vi "Menu.Sequence.Load.vi"(8 "error in (no error)":errorcluster, 9 "Coords":T1, 10 "MenuRef":refnum<k9>, 11 "State Variables":T2={"Aliases.All"=[], "Aliases.Outputs"=[], "UI.Sequence#ofColumns"=0, "SysDef.Path"=path "", "UI.SequenceRef"=refnum, "UI.StepInformationRef"=refnum, "UI.AbortRef"=refnum, "UI.GraphRef"=refnum, "UI.ViewRef"=refnum, "UI.IterationsRef"=refnum, "UI.IterationInformationRef"=refnum, "INI.Settings"={"Build Location"=path "C:/Simple Sequence Editor/SequenceRepo", "LoggingLocation"=path ""}}) -> (0 "error out":errorcluster, 3 "State Variables out":T2={"Aliases.All"=[], "Aliases.Outputs"=[], "UI.Sequence#ofColumns"=0, "SysDef.Path"=path "", "UI.SequenceRef"=refnum, "UI.StepInformationRef"=refnum, "UI.AbortRef"=refnum, "UI.GraphRef"=refnum, "UI.ViewRef"=refnum, "UI.IterationsRef"=refnum, "UI.IterationInformationRef"=refnum, "INI.Settings"={"Build Location"=path "C:/Simple Sequence Editor/SequenceRepo", "LoggingLocation"=path ""}})   [LabVIEW 2013, in "Simple Sequence Tools - Editor.lvlib"]
uses:
  Simple Sequence Tools - Editor.lvlib
  Types/StateVariables.ctl
  Shared/Types/ChannelProperties.ctl
  Shared/Types/INI.Settings
  <vilib>/Utility/miscctls.llb/LVPoint32TypeDef.ctl
  Shared/SubVIs/Constants.vi
  Shared/Simple Sequence Tools - Shared.lvlib
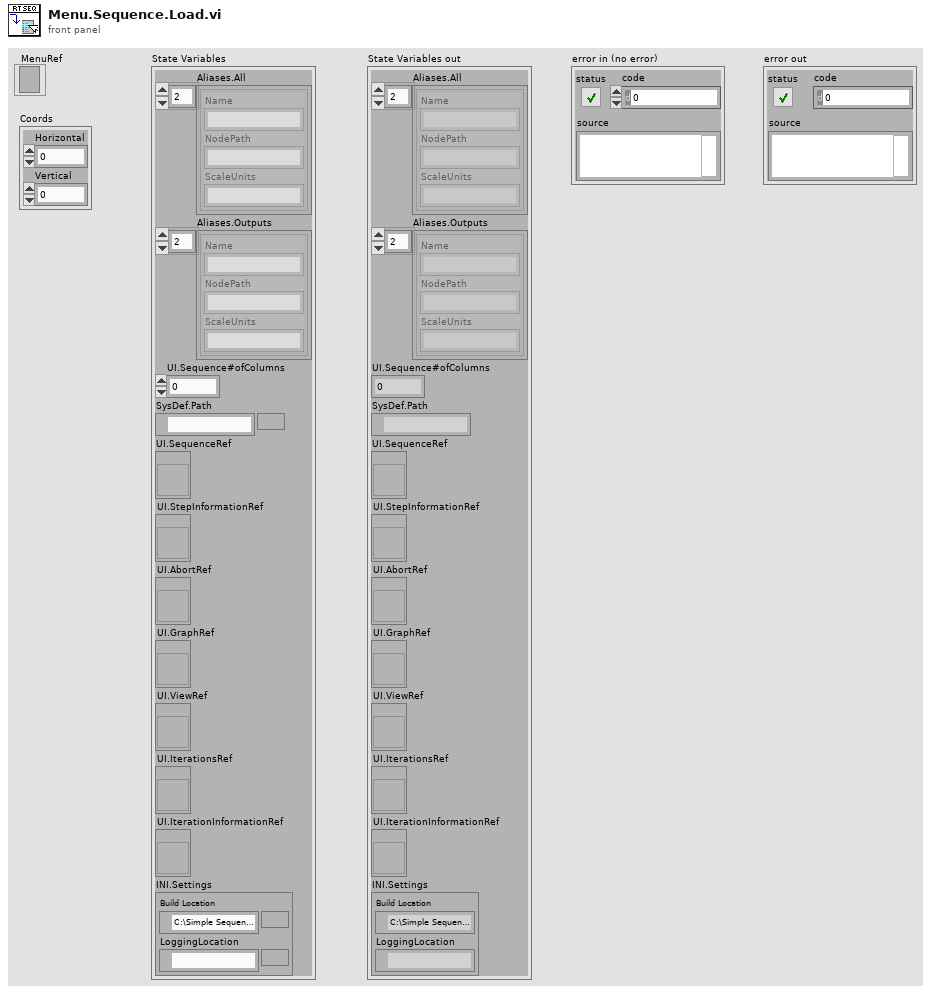
[diagram p1: front panel]
types:
  T1 = typedef "LVPoint32TypeDef.ctl" = cluster{"Horizontal":i32, "Vertical":i32}
  T2 = typedef "Simple Sequence Tools - Editor.lvlib/StateVariables.ctl" = cluster{"Aliases.All":T3[], "Aliases.Outputs":T3[], "UI.Sequence#ofColumns":i32, "SysDef.Path":path, "UI.SequenceRef":refnum<vi>, "UI.StepInformationRef":refnum<vi>, "UI.AbortRef":refnum<vi>, "UI.GraphRef":refnum<vi>, "UI.ViewRef":refnum<vi>, "UI.IterationsRef":refnum<vi>, "UI.IterationInformationRef":refnum<vi>, "INI.Settings":T4}
  T3 = typedef "Simple Sequence Tools - Shared.lvlib/ChannelProperties.ctl" = cluster{"Name":string, "NodePath":string, "ScaleUnits":string}
  T4 = typedef "Simple Sequence Tools - Shared.lvlib/INI.Settings" = cluster{"Build Location":path, "LoggingLocation":path}
  T5 = typedef "LVRowAndColumnTypeDef.ctl" = cluster{"Row":i32, "Column":i32}
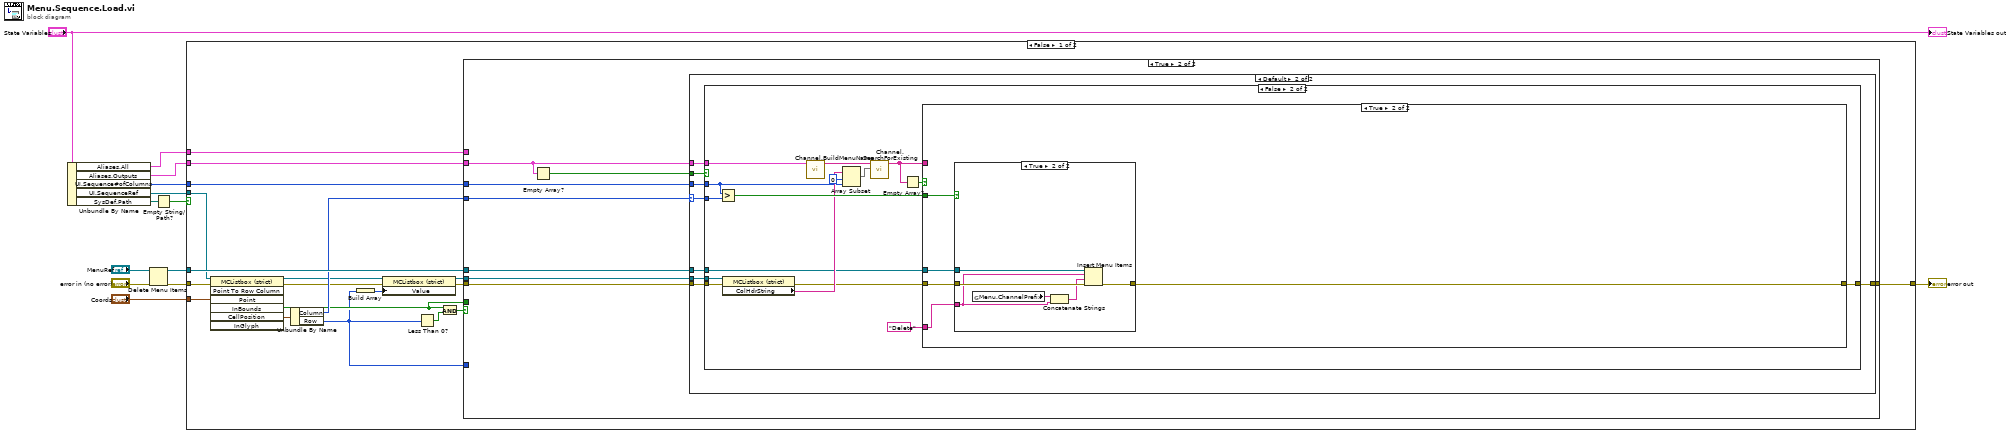
[diagram p0: block diagram]
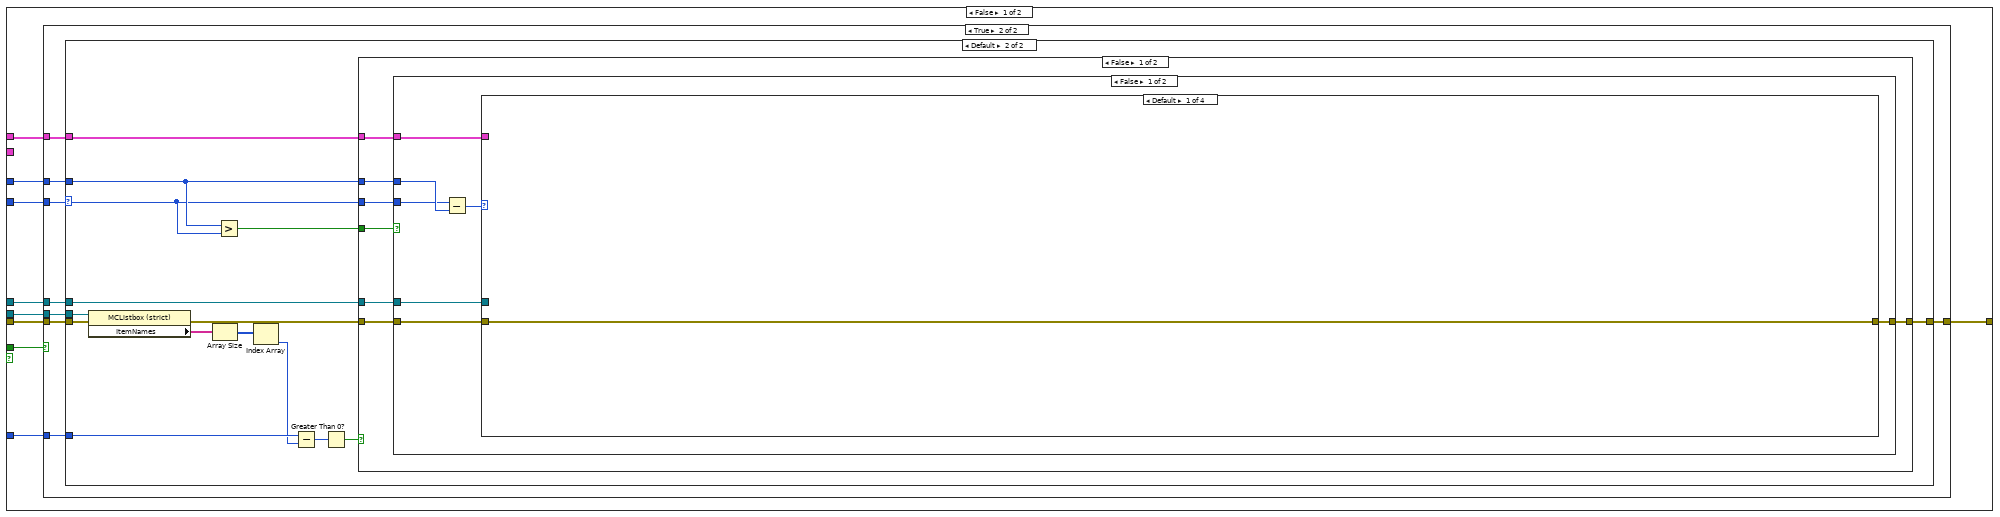
[diagram p2: hidden frame]
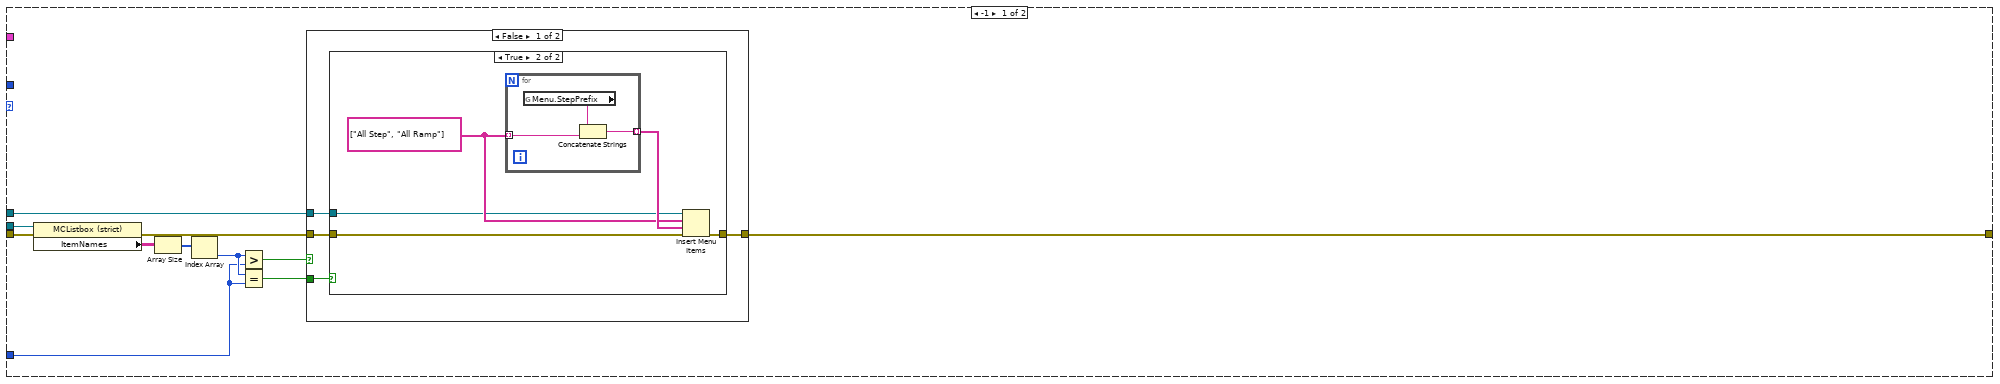
[diagram p4: hidden frame]
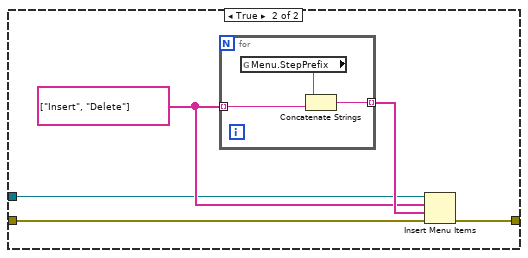
[diagram p6: hidden frame]
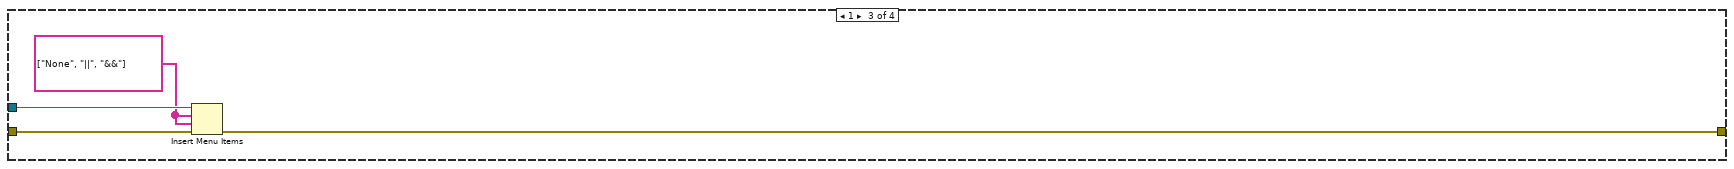
[diagram p8: hidden frame]
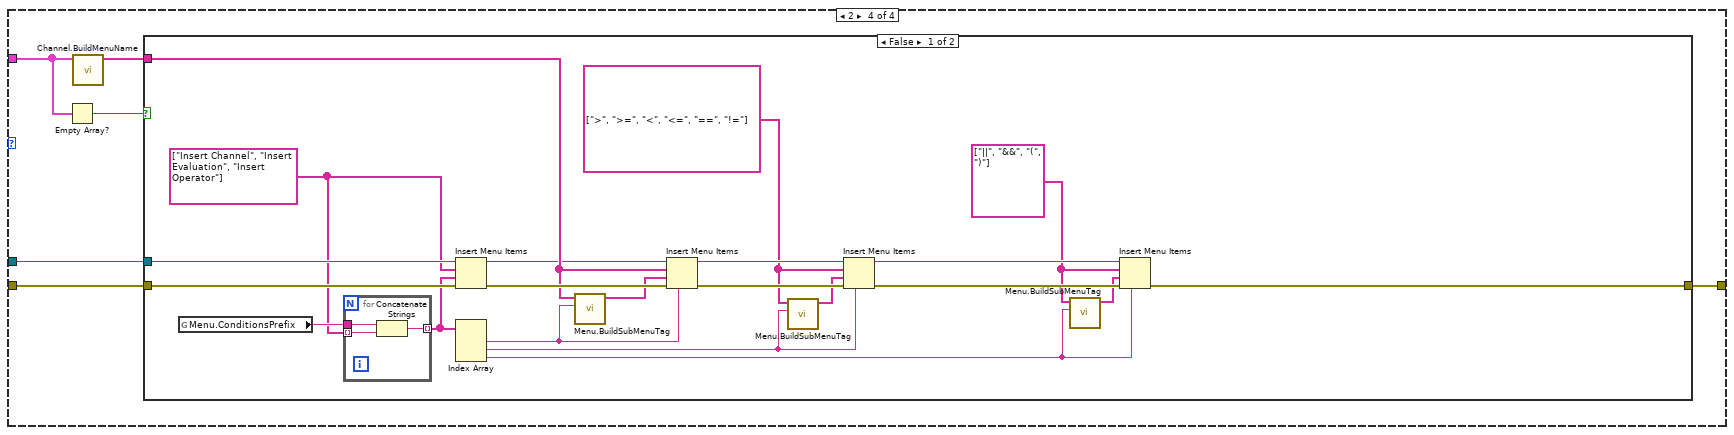
[diagram p9: hidden frame]
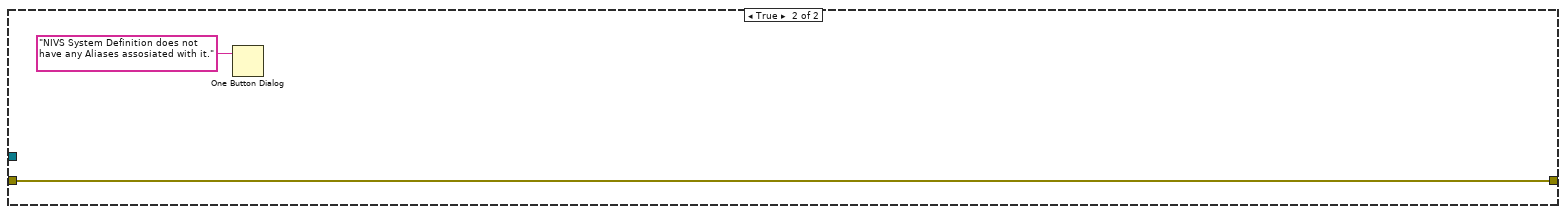
[diagram p10: hidden frame]
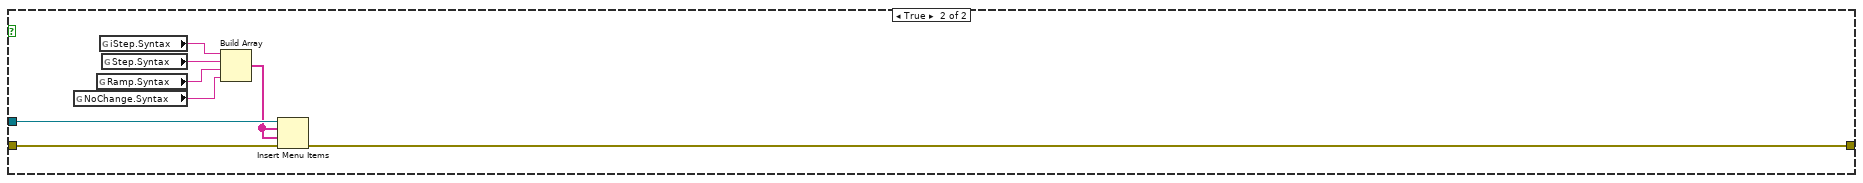
[diagram p11: hidden frame]
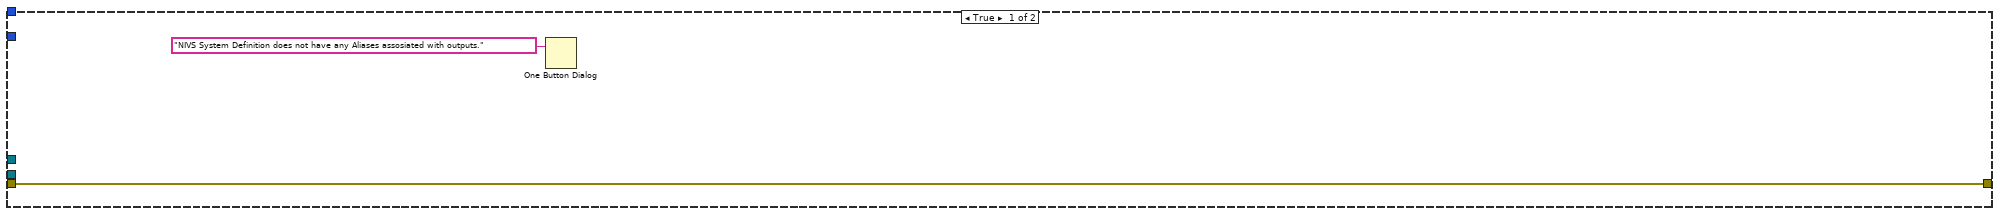
[diagram p14: hidden frame]
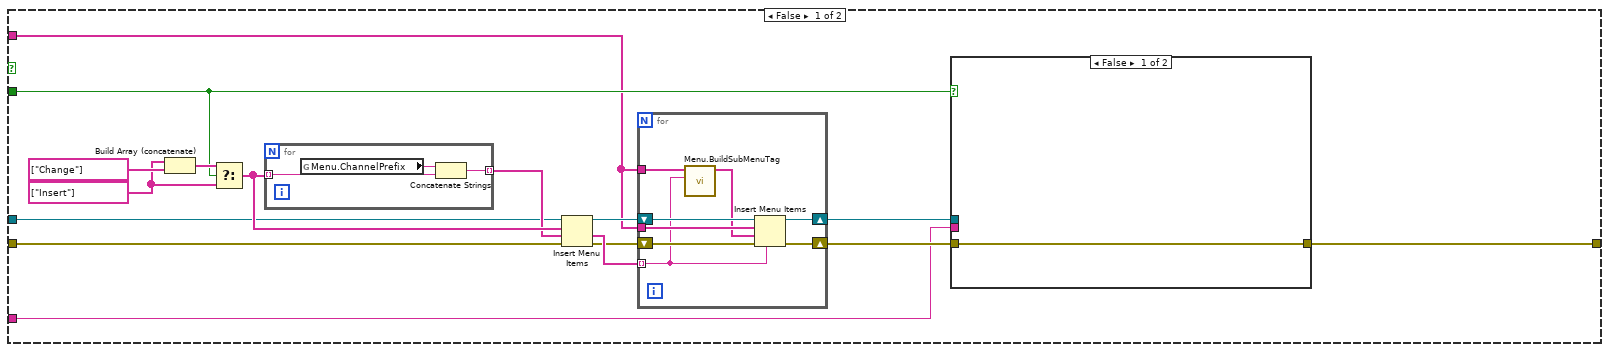
[diagram p15: hidden frame]
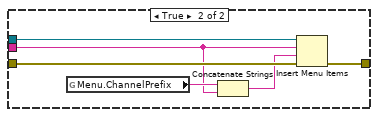
[diagram p16: hidden frame]
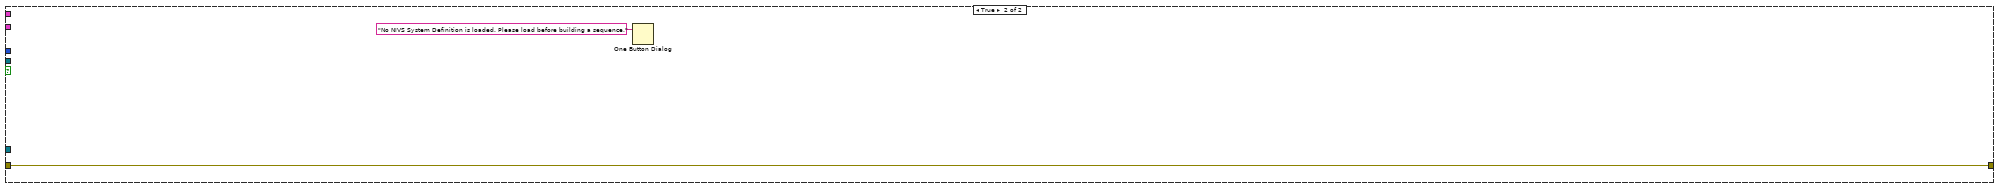
[diagram p18: hidden frame]
diagram:
  n1 = Unbundle By Name("State Variables") -> ("Aliases.All"=w1:T3[], "Aliases.Outputs"=w9:T3[], "UI.Sequence#ofColumns"=w12:i32, "UI.SequenceRef"=w10:refnum<vi>, "SysDef.Path"=w7:path)
  n2 = Delete Menu Items(6:"error in (no error)", 9:"MenuRef") -> (0:w4:errorcluster, 3:w2:refnum<k9>)  [unwired: 2 in]
  n3 = Empty String/Path?(string/path=w7) -> (empty?=w6:bool)
  n4 = case shown="False" w6 {
    tunnel: [w32 w240] -> w13
    tunnel: w2 -> [w31 _]
    tunnel: w12 -> [w30 _]
    tunnel: "Coords" -> [w25 _]
    tunnel: w10 -> [w24 _]
    tunnel: w4 -> [w23 w240]
    tunnel: w9 -> [w22 _]
    tunnel: w1 -> [w20 _]
    frame False {
      n5 = invoke class="MCListbox (strict)" method="Point To Row Column"(reference=w24, error in=w23, "Point"=w25) -> (reference out=w18:refnum<vi>, error out=w19:errorcluster, "InBounds"=w21:bool, "CellPosition"=w26:T5)  [unwired: 4 in, 3 out]
      n6 = Unbundle By Name(w26) -> ("Column"=w29:i32, "Row"=w15:i32)
      n7 = Build Array(w15) -> (w14:i32[])
      n8 = property class="MCListbox (strict)"(reference=w18, error in=w19, "Value"=w14) -> (reference out=w16:refnum<vi>, error out=w17:errorcluster)
      n9 = Less Than 0?(x=w15) -> (x < 0?=w27:bool)
      n10 = And(x=w21, y=w27) -> (x .and. y?=w28:bool)
      n11 = case shown="True" w28 {
        tunnel: w29 -> [w36 w159]
        tunnel: w30 -> [w37 w160]
        tunnel: w31 -> [w35 w163]
        tunnel: w17 -> [w40 w164]
        tunnel: [w34 w165] -> w32
        tunnel: w16 -> [w39 w166]
        tunnel: w22 -> [_ w162]
        tunnel: w21 -> [w41 _]
        tunnel: w15 -> [w38 _]
        tunnel: w20 -> [w33 _]
        frame False {
          n12 = case shown="True" w41 {
            tunnel: w40 -> [w42 w49]
            tunnel: w39 -> [_ w50]
            tunnel: w38 -> [_ w48]
            tunnel: w37 -> [_ w47]
            tunnel: w36 -> [_ w46]
            tunnel: w35 -> [_ w45]
            tunnel: [w42 w44] -> w34
            tunnel: w33 -> [_ w43]
            frame False {
            }
            frame True {
              n13 = case shown="Default" w46 {
                selector: w46 -> [_ w87]
                tunnel: w50 -> [w57 w97]
                tunnel: w49 -> [w59 w96]
                tunnel: w48 -> [w52 w93]
                tunnel: w47 -> [_ w88]
                tunnel: w45 -> [w60 w89]
                tunnel: [w61 w85] -> w44
                tunnel: w43 -> [_ w83]
                frame -1 {
                  n14 = property class="MCListbox (strict)"(reference=w57, error in=w59) -> (error out=w58:errorcluster, "ItemNames"=w55:string[][])  [unwired: 1 out]
                  n15 = Array Size(array=w55) -> (size(s)=w56:i32[])
                  n16 = Index Array(array=w56) -> (element=w53:i32)  [unwired: 1 in]
                  n17 = Greater?(x=w53, y=w52) -> (0:w54:bool)
                  n18 = Equal?(x=w53, y=w52) -> (x = y?=w51:bool)
                  n19 = case shown="False" w54 {
                    tunnel: [w64 w79] -> w61
                    tunnel: w60 -> [w63 w76]
                    tunnel: w58 -> [w65 w75]
                    tunnel: w51 -> [w62 _]
                    frame False {
                      n20 = case shown="True" w62 {
                        tunnel: w65 -> [w66 w69]
                        tunnel: [w66 w68] -> w64
                        tunnel: w63 -> [_ w67]
                        frame False {
                        }
                        frame True {
                          w70 = string[] ["All Step", "All Ramp"] ("item names")
                          n21 = for {
                            tunnel: [w73] -> w71 mode=indexing
                            tunnel: w70 -> [w74] mode=indexing
                            n22 = global read "Constants.vi" "Menu.StepPrefix"() -> (w72:string)
                            n23 = Concatenate Strings(w72, w74) -> (w73:string)
                          }
                          n24 = Insert Menu Items(6:w69, 7:w71, 8:w70, 9:w67) -> (0:w68:errorcluster)  [unwired: 2 in, 2 out]
                        }
                      }
                    }
                    frame True {
                      w77 = string[] ["Insert", "Delete"] ("item names")
                      n25 = for {
                        tunnel: [w81] -> w78 mode=indexing
                        tunnel: w77 -> [w82] mode=indexing
                        n26 = global read "Constants.vi" "Menu.StepPrefix"() -> (w80:string)
                        n27 = Concatenate Strings(w80, w82) -> (w81:string)
                      }
                      n28 = Insert Menu Items(6:w75, 7:w78, 8:w77, 9:w76) -> (0:w79:errorcluster)  [unwired: 2 in, 2 out]
                    }
                  }
                }
                frame Default {
                  n29 = property class="MCListbox (strict)"(reference=w97, error in=w96) -> (error out=w91:errorcluster, "ItemNames"=w95:string[][])  [unwired: 1 out]
                  n30 = Array Size(array=w95) -> (size(s)=w94:i32[])
                  n31 = Greater?(x=w88, y=w87) -> (0:w86:bool)
                  n32 = Index Array(array=w94) -> (element=w92:i32)  [unwired: 1 in]
                  n33 = Subtract(x=w93, y=w92) -> (x-y=w84:i32)
                  n34 = Greater Than 0?(x=w84) -> (x > 0?=w90:bool)
                  n35 = case shown="False" w90 {
                    tunnel: w91 -> [w104 w158]
                    tunnel: w88 -> [w101 _]
                    tunnel: w87 -> [w100 _]
                    tunnel: w89 -> [w103 _]
                    tunnel: w86 -> [w102 _]
                    tunnel: [w99 w158] -> w85
                    tunnel: w83 -> [w98 _]
                    frame False {
                      n36 = case shown="False" w102 {
                        tunnel: w104 -> [w107 w157]
                        tunnel: w103 -> [w108 w155]
                        tunnel: w101 -> [w111 _]
                        tunnel: w100 -> [w110 _]
                        tunnel: [w106 w156] -> w99
                        tunnel: w98 -> [w105 _]
                        frame False {
                          n37 = Subtract(x=w110, y=w111) -> (x-y=w109:i32)
                          n38 = case shown="Default" w109 {
                            tunnel: w108 -> [_ _ w117 w123]
                            tunnel: w107 -> [w112 w113 w116 w122]
                            tunnel: [w112 w113 w114 w121] -> w106
                            tunnel: w105 -> [_ _ _ w120]
                            frame Default {
                            }
                            frame 0 {
                            }
                            frame 1 {
                              w115 = string[] ["None", "||", "&&"] ("item names")
                              n39 = Insert Menu Items(6:w116, 7:w115, 8:w115, 9:w117) -> (0:w114:errorcluster)  [unwired: 2 in, 2 out]
                            }
                            frame 2 {
                              n40 = Empty Array?(array=w120) -> (empty?=w119:bool)
                              n41 = call "Channel.BuildMenuName.vi"("Aliases"=w120) -> ("Aliases Array"=w118:string[])  [unwired: 10 in]
                              n42 = case shown="False" w119 {
                                tunnel: w123 -> [w144 _]
                                tunnel: w122 -> [w143 w148]
                                tunnel: [w132 w148] -> w121
                                tunnel: w118 -> [w138 _]
                                frame False {
                                w125 = string[] [">", ">=", "<", "<=", "==", "!="] ("item names")
                                w124 = string[] ["||", "&&", "(", ")"] ("item names")
                                w141 = string[] ["Insert Channel", "Insert Evaluation", "Insert Operator"] ("item names")
                                n43 = global read "Constants.vi" "Menu.ConditionsPrefix"() -> (w142:string)
                                n44 = for {
                                tunnel: w141 -> [w147] mode=indexing
                                tunnel: w142 -> [w146]
                                tunnel: [w145] -> w135 mode=indexing
                                n45 = Concatenate Strings(w146, w147) -> (w145:string)
                                }
                                n46 = Insert Menu Items(6:w143, 7:w135, 8:w141, 9:w144) -> (0:w140:errorcluster, 3:w137:refnum<k9>)  [unwired: 2 in, 1 out]
                                n47 = Index Array(array=w135) -> (element #1=w136:string, element #2=w129:string, element #3=w127:string)  [unwired: 3 in]
                                n48 = call "Menu.BuildSubMenuTag.vi"("Menu"=w136, "Aliases Array"=w138) -> ("Tag Array"=w139:string[])  [unwired: 9 in]
                                n49 = Insert Menu Items(5:w136, 6:w140, 7:w139, 8:w138, 9:w137) -> (0:w134:errorcluster, 3:w131:refnum<k9>)  [unwired: 1 in, 1 out]
                                n50 = call "Menu.BuildSubMenuTag.vi"("Menu"=w129, "Aliases Array"=w125) -> ("Tag Array"=w128:string[])  [unwired: 9 in]
                                n51 = Insert Menu Items(5:w129, 6:w134, 7:w128, 8:w125, 9:w131) -> (0:w133:errorcluster, 3:w130:refnum<k9>)  [unwired: 1 in, 1 out]
                                n52 = call "Menu.BuildSubMenuTag.vi"("Menu"=w127, "Aliases Array"=w124) -> ("Tag Array"=w126:string[])  [unwired: 9 in]
                                n53 = Insert Menu Items(5:w127, 6:w133, 7:w126, 8:w124, 9:w130) -> (0:w132:errorcluster)  [unwired: 1 in, 2 out]
                                }
                                frame True {
                                n54 = One Button Dialog(message="NIVS System Definition does not have any Aliases assosiated with it.") -> ()  [unwired: 1 in, 1 out]
                                }
                              }
                            }
                          }
                        }
                        frame True {
                          n55 = global read "Constants.vi" "NoChange.Syntax"() -> (w151:string)
                          n56 = global read "Constants.vi" "Ramp.Syntax"() -> (w153:string)
                          n57 = global read "Constants.vi" "iStep.Syntax"() -> (w150:string)
                          n58 = global read "Constants.vi" "Step.Syntax"() -> (w154:string)
                          n59 = Build Array(w150, w154, w153, w151) -> (w152:string[])
                          n60 = Insert Menu Items(6:w157, 7:w152, 8:w152, 9:w155) -> (0:w156:errorcluster)  [unwired: 2 in, 2 out]
                        }
                      }
                    }
                    frame True {
                    }
                  }
                }
              }
            }
          }
        }
        frame True {
          n61 = Empty Array?(array=w162) -> (empty?=w161:bool)
          n62 = case shown="Default" w159 {
            selector: w159 -> [_ w168]
            tunnel: w166 -> [_ w175]
            tunnel: [w167 w174] -> w165
            tunnel: w164 -> [w167 w173]
            tunnel: w163 -> [_ w172]
            tunnel: w162 -> [_ w171]
            tunnel: w161 -> [_ w170]
            tunnel: w160 -> [_ w169]
            frame -1 {
            }
            frame Default {
              n63 = case shown="False" w170 {
                tunnel: w168 -> [_ w193]
                tunnel: w175 -> [_ w191]
                tunnel: w169 -> [_ w189]
                tunnel: [w177 w187] -> w174
                tunnel: w171 -> [_ w186]
                tunnel: w173 -> [w177 w182]
                tunnel: w172 -> [_ w183]
                frame True {
                  n64 = One Button Dialog(message="NIVS System Definition does not have any Aliases assosiated with outputs.") -> ()  [unwired: 1 in, 1 out]
                }
                frame False {
                  n65 = Greater?(x=w189, y=w193) -> (0:w192:bool)
                  n66 = property class="MCListbox (strict)"(reference=w191, error in=w182) -> (error out=w181:errorcluster, "ColHdrString"=w190:string[])  [unwired: 1 out]
                  n67 = call "Channel.BuildMenuName.vi"("Aliases"=w186) -> ("Aliases Array"=w184:string[])  [unwired: 10 in]
                  n68 = Array Subset(array=w190, index=0, length=w189) -> (w185:string[])
                  n69 = call "Channel.SearchForExisting.vi"("Existing Channels"=w185, "All Channels"=w184) -> ("Array out"=w180:string[])  [unwired: 9 in]
                  n70 = Empty Array?(array=w180) -> (empty?=w179:bool)
                  n71 = case shown="True" w179 {
                    tunnel: w192 -> [w195 w228]
                    tunnel: [w198 w231] -> w187
                    tunnel: w183 -> [w202 w230]
                    tunnel: w180 -> [w194 _]
                    tunnel: w181 -> [w200 w232]
                    tunnel: "Delete" ("string") -> [w196 w229]
                    frame False {
                      w207 = string[] ["Insert"]
                      n72 = Build Array (concatenate)(w207, string[] ["Change"]) -> (w208:string[])
                      n73 = Select(t=w208, s=w195, f=w207) -> (s? t:f=w206:string[])
                      n74 = for {
                        tunnel: w206 -> [w227] mode=indexing
                        tunnel: [w226] -> w205 mode=indexing
                        n75 = global read "Constants.vi" "Menu.ChannelPrefix"() -> (w225:string)
                        n76 = Concatenate Strings(w225, w227) -> (w226:string)
                      }
                      n77 = Insert Menu Items(6:w200, 7:w205, 8:w206, 9:w202) -> (0:w201:errorcluster, 1:w203:string[], 3:w204:refnum<k9>)  [unwired: 2 in]
                      n78 = for {
                        tunnel: w203 -> [w219] mode=indexing
                        shift-right: [w223] -> w199
                        shift-left: w201 -> [w224]
                        tunnel: w194 -> [w221]
                        shift-right: [w220] -> w197
                        shift-left: w204 -> [w222]
                        tunnel: w194 -> [w218]
                        n79 = call "Menu.BuildSubMenuTag.vi"("Menu"=w219, "Aliases Array"=w218) -> ("Tag Array"=w217:string[])  [unwired: 9 in]
                        n80 = Insert Menu Items(5:w219, 6:w224, 7:w217, 8:w221, 9:w222) -> (0:w223:errorcluster, 3:w220:refnum<k9>)  [unwired: 1 in, 1 out]
                      }
                      n81 = case shown="False" w195 {
                        tunnel: w199 -> [w210 w216]
                        tunnel: [w210 w215] -> w198
                        tunnel: w197 -> [_ w214]
                        tunnel: w196 -> [_ w211]
                        frame False {
                        }
                        frame True {
                          n82 = global read "Constants.vi" "Menu.ChannelPrefix"() -> (w213:string)
                          n83 = Concatenate Strings(w213, w211) -> (w212:string)
                          n84 = Insert Menu Items(6:w216, 7:w212, 8:w211, 9:w214) -> (0:w215:errorcluster)  [unwired: 2 in, 2 out]
                        }
                      }
                    }
                    frame True {
                      n85 = case shown="True" w228 {
                        tunnel: w232 -> [w233 w239]
                        tunnel: [w233 w238] -> w231
                        tunnel: w230 -> [_ w237]
                        tunnel: w229 -> [_ w235]
                        frame False {
                        }
                        frame True {
                          n86 = global read "Constants.vi" "Menu.ChannelPrefix"() -> (w236:string)
                          n87 = Concatenate Strings(w236, w235) -> (w234:string)
                          n88 = Insert Menu Items(6:w239, 7:w234, 8:w235, 9:w237) -> (0:w238:errorcluster)  [unwired: 2 in, 2 out]
                        }
                      }
                    }
                  }
                }
              }
            }
          }
        }
      }
    }
    frame True {
      n89 = One Button Dialog(message="No NIVS System Definition is loaded. Please load before building a sequence.") -> ()  [unwired: 1 in, 1 out]
    }
  }
  "error out" <- w13
  "State Variables out" <- "State Variables"
